vi "MainInterfacePCloop.vi"() -> ()   [LabVIEW 2015]
panel:
  out "Waveform Graph 2":i32[](graph)
  out "SampleStartTime":dbl
  out "run time (ms)":u32
  out "float image":T1(plugin-control)
  out "Index":i32
  in  "Stop Button":bool
  out "loop index":i32
  in  "ICImagingControl":refnum<k7>(container)
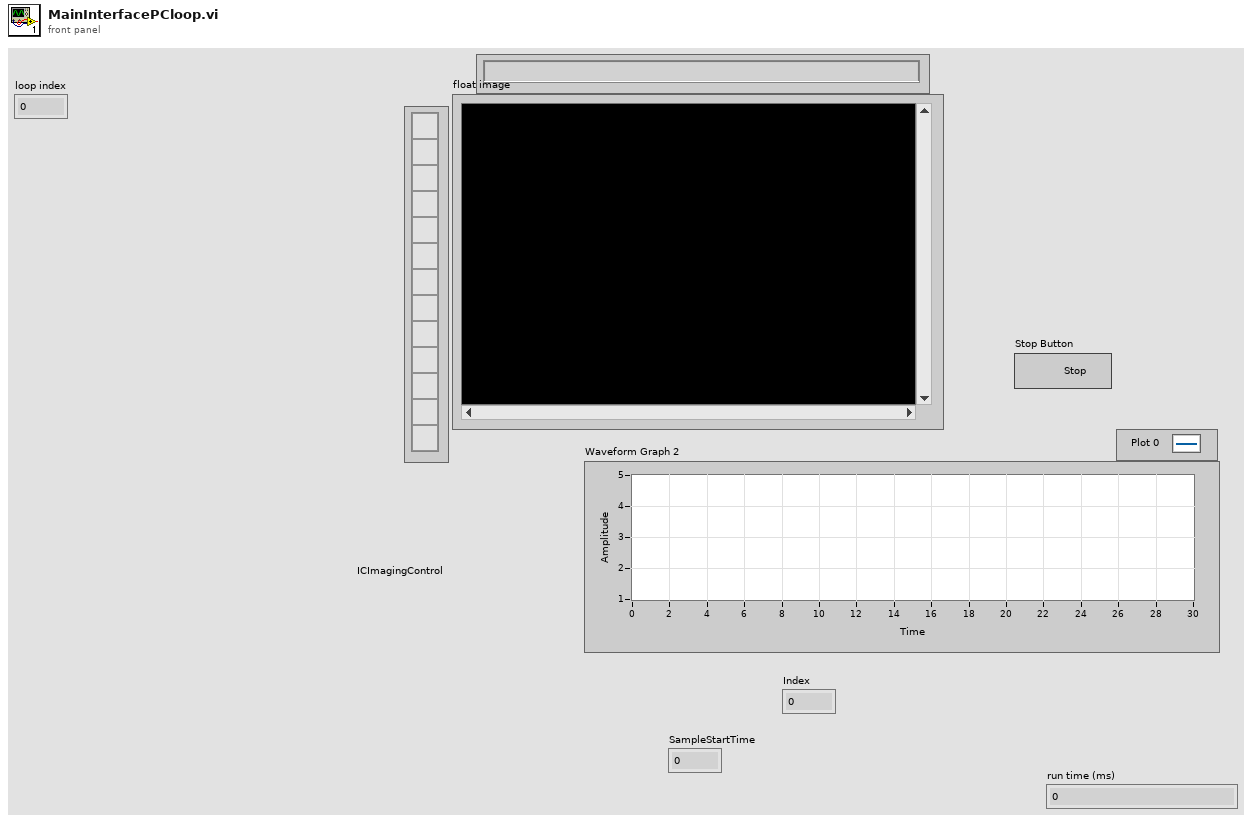
[diagram p1: front panel]
types:
  T1 = typedef "IMAQ Image.ctl" = refnum<image>
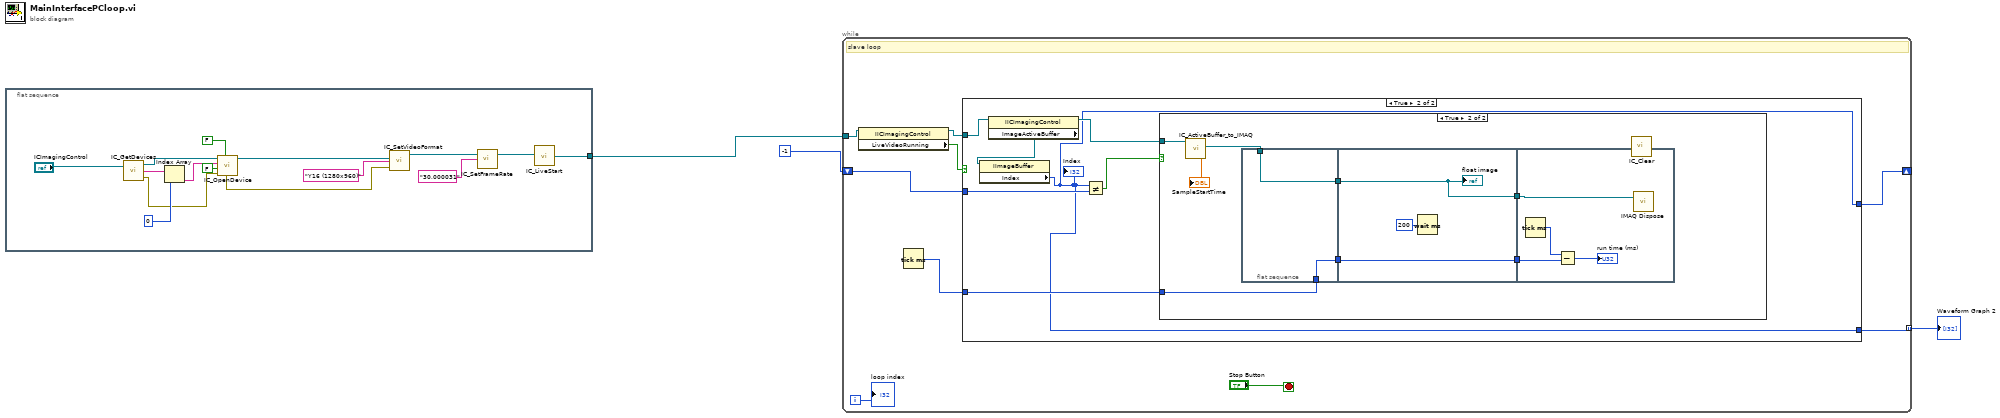
[diagram p0: block diagram]
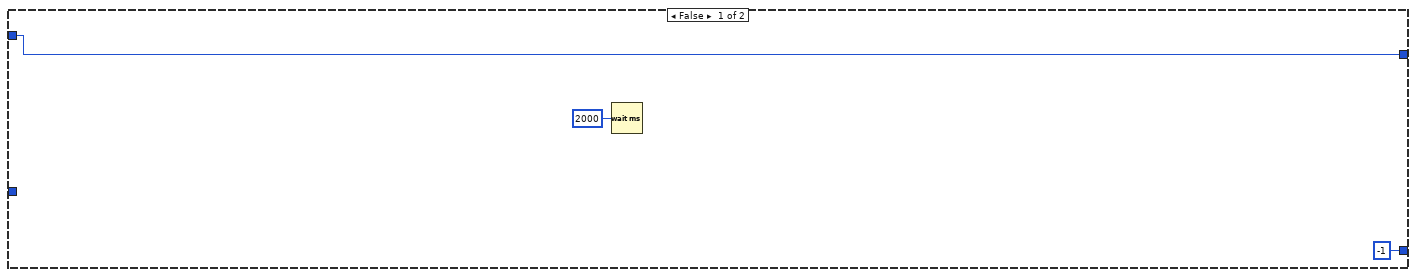
[diagram p2: hidden frame]
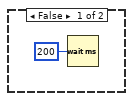
[diagram p3: hidden frame]
diagram:
  n1 = flat-sequence {
    tunnel: [w7] -> w1
    frame #0 {
      n2 = call <userlib>:"IC_GetDevices.vi"("ICImagingControl In"="ICImagingControl") -> ("ICImagingControl Out"=w15:refnum<k7>, "Devices"=w17:string[], "Error Out"=w12:errorcluster)  [unwired: 1 in]
      n3 = Index Array(array=w17, index=0) -> (element=w14:string)
      n4 = call <userlib>:"IC_OpenDevice.vi"("Color"=FALSE, "Error In (no error)"=w12, "Live"=FALSE, "Device"=w14, "ICImagingControl In"=w15) -> ("ICImagingControl Out"=w11:refnum<k7>, "Error Out"=w8:errorcluster)  [unwired: 1 in, 4 out]
      n5 = call <userlib>:"IC_SetVideoFormat.vi"("Error In (no error)"=w8, "VideoFormat"="Y16 (1280x960)", "ICImagingControl In"=w11) -> ("ICImagingControl Out"=w10:refnum<k7>)  [unwired: 2 out]
      n6 = call <userlib>:"IC_SetFrameRate.vi"("FrameRate"="30,000031", "ICImagingControl In"=w10) -> ("ICImagingControl Out"=w6:refnum<k7>)  [unwired: 1 in, 1 out]
      n7 = call <userlib>:"IC_LiveStart.vi"("ICImagingControl 3"=w6) -> ("ICImagingControl 2"=w7:refnum<k7>)
    }
  }
  n8 = while {
    tunnel: w1 -> [w26]
    shift-right: [w22] -> _
    shift-left: -1 ("Index") -> [w27]
    tunnel: [w19] -> w2 mode=indexing
    i -> [w20]
    stop <- "Stop Button" stop-if-true
    # "slave loop"
    n9 = property class="IICImagingControl"(reference=w26) -> (reference out=w25:refnum<k7>, "LiveVideoRunning"=w24:bool)  [unwired: 1 in, 1 out]
    n10 = Tick Count (ms)() -> (millisecond timer value=w21:u32)
    n11 = case shown="True" w24 {
      tunnel: w27 -> [w30 w37]
      tunnel: w25 -> [_ w36]
      tunnel: [w30 w32] -> w22
      tunnel: w21 -> [_ w33]
      tunnel: [-1 ("Index") w32] -> w19
      frame False {
        n12 = Wait (ms)(milliseconds to wait=u32 2000) -> ()  [unwired: 1 out]
      }
      frame True {
        n13 = property class="IICImagingControl"(reference=w36) -> (reference out=w34:refnum<k7>, "ImageActiveBuffer"=w35:refnum<k7>)  [unwired: 1 in, 1 out]
        n14 = property class="IImageBuffer"(reference=w35) -> ("Index"=w32:i32)  [unwired: 1 in, 2 out]
        "Index" <- w32
        n15 = Not Equal?(x=w32, y=w37) -> (x != y?=w31:bool)
        n16 = case shown="True" w31 {
          tunnel: w34 -> [_ w46]
          tunnel: w33 -> [_ w40]
          frame False {
            n17 = Wait (ms)(milliseconds to wait=u32 200) -> ()  [unwired: 1 out]
          }
          frame True {
            n18 = call <userlib>:"IC_ActiveBuffer_to_IMAQ.vi"("ICImagingControl In"=w46) -> ("Image Out"=w44:T1, "SampleStartTime"=→"SampleStartTime":dbl)  [unwired: 2 in, 2 out]
            n19 = flat-sequence {
              tunnel: w44 -> [w48]
              tunnel: [w48] -> w43
              tunnel: [w47] -> w42
              tunnel: w40 -> [w47]
              tunnel: w43 -> [w50]
              tunnel: [w51] -> w41
              tunnel: w42 -> [w51]
              tunnel: [w50] -> w39
              tunnel: w41 -> [w54]
              tunnel: w39 -> [w52]
              frame #0 {
              }
              frame #1 {
                n20 = Wait (ms)(milliseconds to wait=u32 200) -> ()  [unwired: 1 out]
                "float image" <- w50
              }
              frame #2 {
                n21 = Tick Count (ms)() -> (millisecond timer value=w55:u32)
                n22 = Subtract(x=w55, y=w54) -> (x-y=→"run time (ms)":u32)
                n23 = call "IMAQ Dispose"("Image"=w52) -> ()  [unwired: 5 in, 1 out]
              }
            }
          }
        }
      }
    }
    "loop index" <- w20
  }
  "Waveform Graph 2" <- w2
  n24 = call <userlib>:"IC_Clear.vi"() -> ()  [unwired: 1 in, 1 out]
